vi "adjust.vi"(8 "error in (no error)":errorcluster, 11 "LightSourceMH110125Tsunami in":refnum<class "LightSourceMH110125Tsunami.lvclass">) -> (0 "error out":errorcluster, 3 "LightSourceMH110125Tsunami out":refnum<class "LightSourceMH110125Tsunami.lvclass">)   [LabVIEW 2010, in "LightSourceMH110125Tsunami.lvclass"]
uses:
  LightSourceMH110125Tsunami.lvclass
  LightSourceMH110125Tsunami.lvclass/LightSourceMH110125Tsunami.ctl
panel:
  in  "power in":dbl[unit](slide) scale=0.0..10.0
  in  "stop":bool
  in  "shutter":bool
  in  "switch off":bool
  in  "initialise?":bool
  out "power":dbl[unit](slide) scale=0.0..10.0
  # "laser"
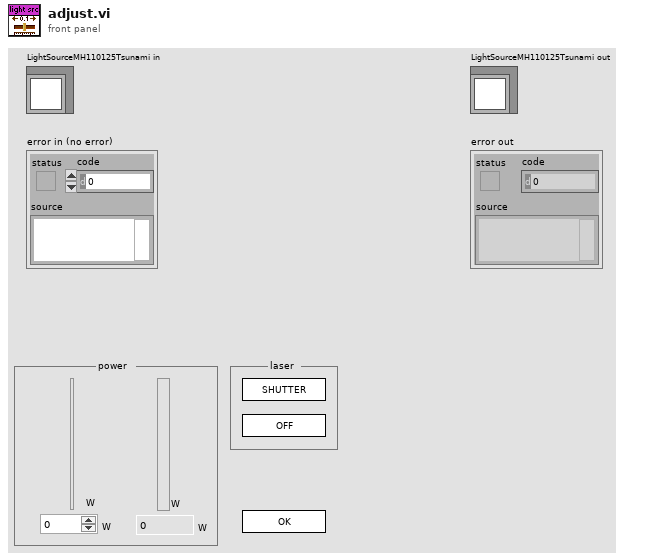
[diagram p1: front panel]
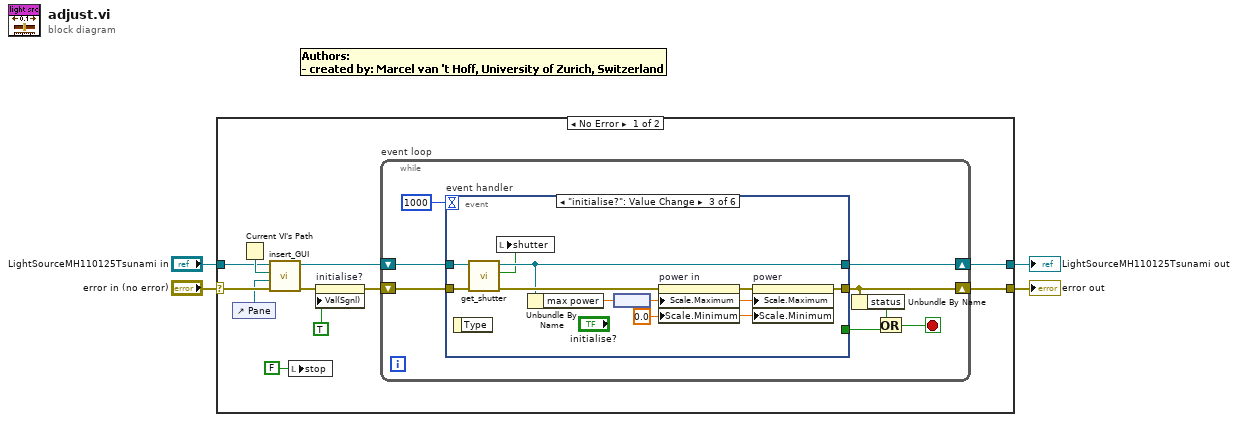
[diagram p0: block diagram]
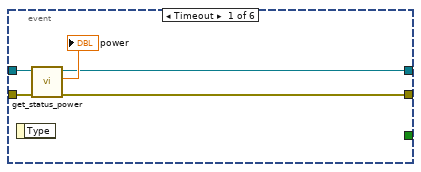
[diagram p2: hidden frame]
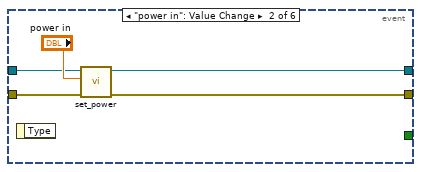
[diagram p3: hidden frame]
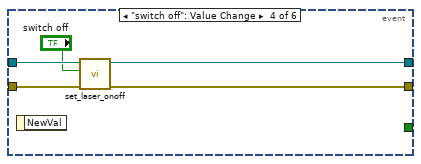
[diagram p4: hidden frame]
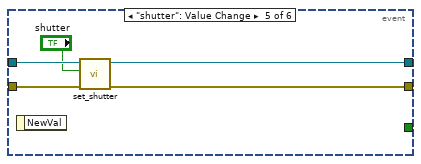
[diagram p5: hidden frame]
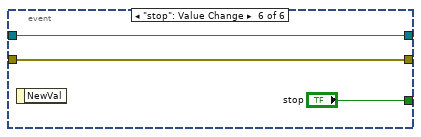
[diagram p6: hidden frame]
diagram:
  n1 = case shown="No Error" "error in (no error)" {
    selector: "error in (no error)" -> [w11 w58]
    tunnel: [w14 w58] -> w2
    tunnel: [w15 w57] -> w1
    tunnel: "LightSourceMH110125Tsunami in" -> [w12 w57]
    frame No Error {
      n2 = control-ref of="Pane"() -> (w5:refnum<vi>)
      n3 = Current VI's Path() -> (path=w13:path)
      n4 = call-dynamic "insert_GUI.vi"("error in (no error)"=w11, "Pane"=w5, "VI path"=w13, "GenericComponent in"=w12) -> ("error out"=w9:errorcluster, "GenericComponent out"=w7:refnum<class "LightSourceMH110125Tsunami.lvclass">)  [unwired: 6 in]
      n5 = local write "stop"(FALSE ("stop")) -> ()
      n6 = property on="initialise?" class="Bool (strict)"(error in=w9, "Val(Sgnl)"=TRUE ("stop")) -> (error out=w8:errorcluster)  [unwired: 1 in, 1 out]
      n7 = while "event loop" {
        shift-right: [w20] -> w14
        shift-left: w8 -> [w21]
        shift-right: [w23] -> w15
        shift-left: w7 -> [w22]
        stop <- w18 stop-if-true
        n8 = event "event handler" shown="[2] \"initialise?\": Value Change" {
          selector: _ -> [_ _ _ _ _ _]
          dyn-events: _ -> [_ _ _ _ _ _]
          timeout: 1000 -> [_ _ _ _ _ _]
          tunnel: [w25 w29 w38 w47 w50 w56] -> w23
          tunnel: w22 -> [w27 w32 w43 w48 w53 w56]
          tunnel: [w24 w30 w39 w46 w49 w55] -> w20
          tunnel: w21 -> [w26 w31 w42 w45 w52 w55]
          tunnel: [_ _ _ _ _ "stop"] -> w17
          event Timeout {
            n9 = event-data() -> ()  [unwired: 1 in, 1 out]
            n10 = call-dynamic "get_status_power.vi"("error in (no error)"=w26, "LightSourceMH110125Tsunami in"=w27) -> ("error out"=w24:errorcluster, "output power"=→"power":dbl[unit], "LightSourceMH110125Tsunami out"=w25:refnum<class "LightSourceMH110125Tsunami.lvclass">)  [unwired: 7 in]
          }
          event "power in": Value Change {
            n11 = event-data() -> ()  [unwired: 1 in, 1 out]
            n12 = call-dynamic "set_power.vi"("error in (no error)"=w31, "power in"="power in", "LightSourceMH110125Tsunami in"=w32) -> ("error out"=w30:errorcluster, "LightSourceMH110125Tsunami out"=w29:refnum<class "LightSourceMH110125Tsunami.lvclass">)  [unwired: 7 in]
          }
          event "initialise?": Value Change {
            w34 = 0.0 ("Scale.Range:Minimum")
            n13 = event-data() -> ()  [unwired: 1 in, 1 out]
            n14 = call-dynamic "get_shutter.vi"("error in (no error)"=w42, "LightSourceMH110125Tsunami in"=w43) -> ("error out"=w41:errorcluster, "shutter open out?"=w36:bool, "LightSourceMH110125Tsunami out"=w38:refnum<class "LightSourceMH110125Tsunami.lvclass">)  [unwired: 7 in]
            n15 = local write "shutter"(w36) -> ()
            n16 = Unbundle By Name(w38) -> ("max power"=w37:dbl[unit])
            n17 = node(w37) -> (w35:dbl)
            n18 = property on="power in" class="Slide (strict)"(error in=w41, "Scale.Maximum"=w35, "Scale.Minimum"=w34) -> (error out=w40:errorcluster)  [unwired: 1 in, 1 out]
            n19 = property on="power" class="Slide (strict)"(error in=w40, "Scale.Maximum"=w35, "Scale.Minimum"=w34) -> (error out=w39:errorcluster)  [unwired: 1 in, 1 out]
          }
          event "switch off": Value Change {
            n20 = event-data() -> ()  [unwired: 1 in, 1 out]
            n21 = call-dynamic "set_laser_onoff.vi"("error in (no error)"=w45, "on?"="switch off", "LightSourceMH110125Tsunami in"=w48) -> ("error out"=w46:errorcluster, "LightSourceMH110125Tsunami out"=w47:refnum<class "LightSourceMH110125Tsunami.lvclass">)  [unwired: 7 in]
          }
          event "shutter": Value Change {
            n22 = event-data() -> ()  [unwired: 1 in, 1 out]
            n23 = call-dynamic "set_shutter.vi"("error in (no error)"=w52, "shutter open?"="shutter", "LightSourceMH110125Tsunami in"=w53) -> ("error out"=w49:errorcluster, "LightSourceMH110125Tsunami out"=w50:refnum<class "LightSourceMH110125Tsunami.lvclass">)  [unwired: 6 in, 1 out]
          }
          event "stop": Value Change {
            n24 = event-data() -> ()  [unwired: 1 in, 1 out]
          }
        }
        n25 = Unbundle By Name(w20) -> ("status"=w19:bool)
        n26 = Or(x=w19, y=w17) -> (x .or. y?=w18:bool)
      }
    }
    frame Error {
    }
  }
  "error out" <- w2
  "LightSourceMH110125Tsunami out" <- w1
